vi "Hardware Scan.vi"(8 "error in (no error)":errorcluster, 11 "Controller in":refnum<class "Controller.lvclass">) -> (0 "error out":errorcluster, 3 "Controller out":refnum<class "Controller.lvclass">)   [LabVIEW 2016, in "Controller Actor.lvlib" / "Controller.lvclass"]
uses:
  Controller.lvclass
  Hardware/Hardware.lvclass
  Controller.lvclass/Controller.ctl
  Accessors/Read Root Path.vi
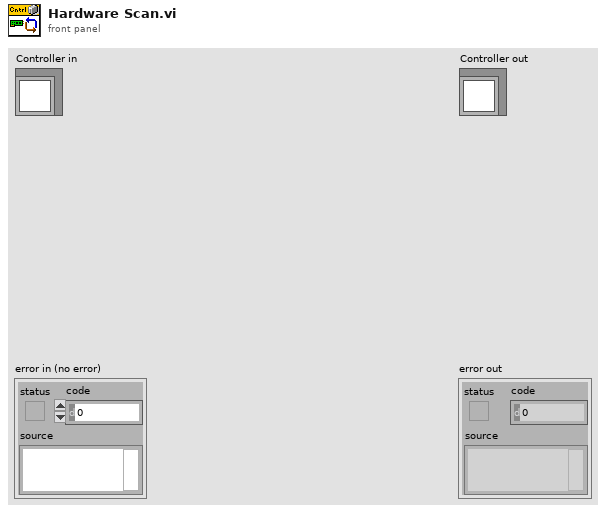
[diagram p1: front panel]
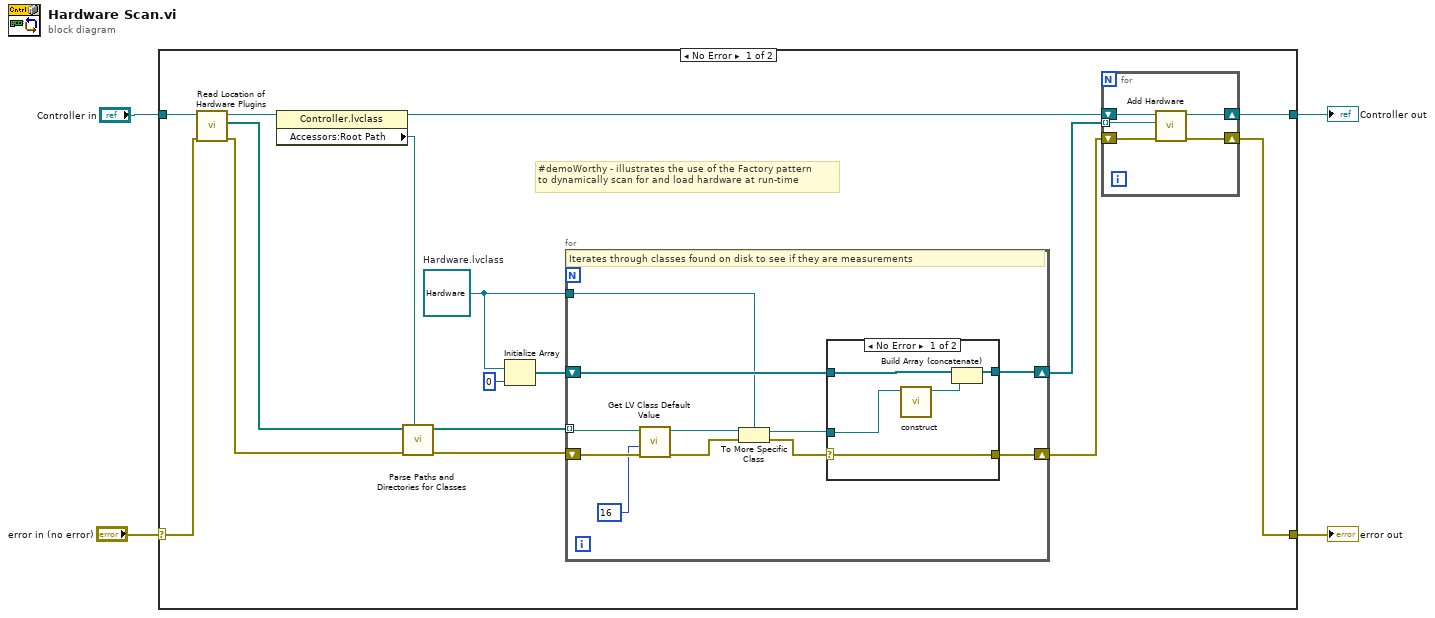
[diagram p0: block diagram]
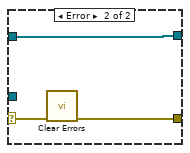
[diagram p2: hidden frame]
diagram:
  n1 = case shown="No Error" "error in (no error)" {
    selector: "error in (no error)" -> [w14 w46]
    tunnel: [w13 w46] -> w3
    tunnel: [w20 w45] -> w1
    tunnel: "Controller in" -> [w19 w45]
    frame No Error {
      w17 = refnum<class "Hardware.lvclass"> refnum  # Hardware.lvclass
      # "#demoWorthy - illustrates the use of the Factory pattern\nto dynamically scan for and load hardware at run-time"
      n2 = call "Read Location of Hardware Plugins.vi"("error in (no error)"=w14, "Controller in"=w19) -> ("error out"=w11:errorcluster, "Array of Hardware Paths"=w12:path[], "Controller out"=w7:refnum<class "Controller.lvclass">)  [unwired: 7 in]
      n3 = property class="Controller.lvclass"(reference=w7) -> (reference out=w5:refnum<class "Controller.lvclass">, "Accessors:Root Path"=w6:path)  [unwired: 1 in, 1 out]
      n4 = call "Parse Paths and Directories for Classes.vi"("base path"=w6, "error in (no error)"=w11, "Array of paths (folders to scan or explicit files)"=w12) -> ("error out"=w10:errorcluster, "All Files in Dir"=w9:path[])  [unwired: 7 in]
      n5 = Initialize Array(w17, 0 ("dimension size")) -> (w16:refnum<class "Hardware.lvclass">[])
      n6 = for {
        tunnel: w9 -> [w30] mode=indexing
        shift-right: [w35] -> w18
        shift-left: w16 -> [w32]
        shift-right: [w31] -> w8
        shift-left: w10 -> [w33]
        tunnel: w17 -> [w28]
        # "Iterates through classes found on disk to see if they are measurements"
        n7 = call <vilib>:"Get LV Class Default Value.vi"("error in (no error)"=w33, "options"=u32 16, "class path"=w30) -> ("error out"=w34:errorcluster, "object"=w29:refnum<class>)  [unwired: 7 in]
        n8 = To More Specific Class(target class=w28, reference=w29, error in=w34) -> (specific class reference=w36:refnum<class "Hardware.lvclass">, error out=w27:errorcluster)
        n9 = case shown="No Error" w27 {
          selector: w27 -> [w40 w43]
          tunnel: w36 -> [w38 _]
          tunnel: [w39 w44] -> w35
          tunnel: w32 -> [w41 w44]
          tunnel: [w40 w42] -> w31
          frame No Error {
            n10 = call-dynamic "construct.vi"("Hardware in"=w38) -> ("Hardware out"=w37:refnum<class "Hardware.lvclass">)  [unwired: 9 in, 1 out]
            n11 = Build Array (concatenate)(w41, w37) -> (w39:refnum<class "Hardware.lvclass">[])
          }
          frame Error {
            n12 = call <vilib>:"Clear Errors.vi"("error in (no error)"=w43) -> ("error out"=w42:errorcluster)  [unwired: 5 in, 1 out]
          }
        }
      }
      n13 = for {
        shift-right: [w24] -> w20
        shift-left: w5 -> [w25]
        tunnel: w18 -> [w23] mode=indexing
        shift-right: [w21] -> w13
        shift-left: w8 -> [w22]
        n14 = call "Add Hardware.vi"("error in (no error)"=w22, "Hardware.lvclass"=w23, "Controller in"=w25) -> ("error out"=w21:errorcluster, "Controller out"=w24:refnum<class "Controller.lvclass">)  [unwired: 7 in]
      }
    }
    frame Error {
    }
  }
  "error out" <- w3
  "Controller out" <- w1
